vi "Fake Resolve Service.vi"(8 "error in":errorcluster, 11 "resolve service request":T1) -> (0 "error out":errorcluster, 3 "service location":T2)   [LabVIEW 2020, in "MeasurementServerTests.lvlib" / "Discovery Tests.lvlib"]
uses:
  Discovery Tests.lvlib
  gRPC/Generated APIs/ni/measurementlink/discovery/v1/RPC Messages/ni_measurementlink_discovery_v1_ServiceLocation.ctl
  gRPC/Generated APIs/ni/measurementlink/discovery/v1/ni.measurementlink.discovery.v1.lvlib
  gRPC/Generated APIs/ni/measurementlink/discovery/v1/RPC Messages/ni_measurementlink_discovery_v1_ResolveServiceRequest.ctl
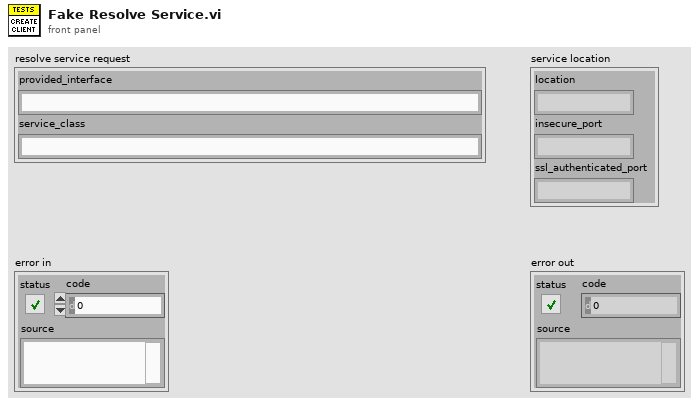
[diagram p1: front panel]
types:
  T1 = typedef "ni.measurementlink.discovery.v1.lvlib/ni_measurementlink_discovery_v1_ResolveServiceRequest.ctl" = cluster{"provided_interface":string, "service_class":string}
  T2 = typedef "ni.measurementlink.discovery.v1.lvlib/ni_measurementlink_discovery_v1_ServiceLocation.ctl" = cluster{"location":string, "insecure_port":string, "ssl_authenticated_port":string}
  T3 = typedef "Measurement Plugin Discovery Client.lvlib/ni_measurementlink_discovery_v1_ServiceLocation.ctl" = cluster{"location":string, "insecure_port":string, "ssl_authenticated_port":string}
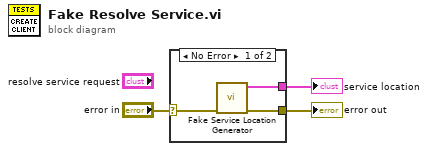
[diagram p0: block diagram]
diagram:
  n1 = case shown="No Error" "error in" {
    selector: "error in" -> [w6 w7]
    tunnel: [w5 w7] -> w2
    tunnel: [w4 _] -> w1
    frame No Error {
      n2 = call "Fake Service Location Generator.vi"("error in"=w6) -> ("error out"=w5:errorcluster, "service location"=w4:T3)  [unwired: 9 in]
    }
    frame Error {
    }
  }
  "error out" <- w2
  "service location" <- w1
